vi "CRYFlatten Data Read.vi"(6 "error in":errorcluster, 9 "Path In":path) -> (0 "error out":errorcluster, 2 "Flatten Data Out":string, 3 "Path Out":path)   [LabVIEW 2013]
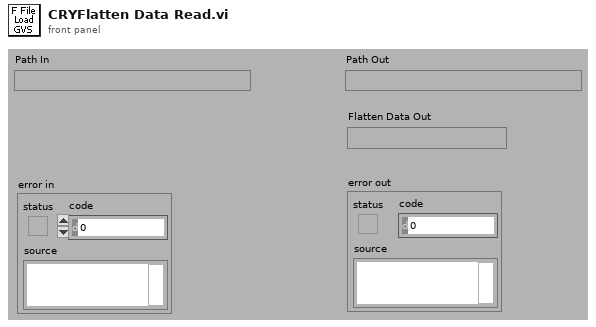
[diagram p1: front panel]
types:
  T1 = enum16{"open", "replace", "create", "open or create", "replace or create", "replace or create with confirmation"}
  T2 = enum16{"big-endian, network order", "native, host order", "little-endian"}
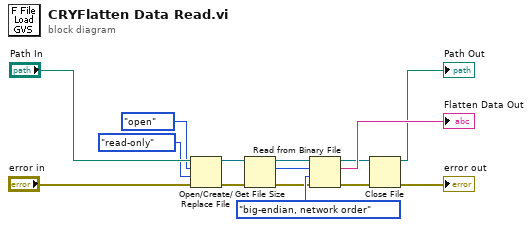
[diagram p0: block diagram]
diagram:
  n1 = Open/Create/Replace File(file path (use dialog)="Path In", error in="error in", operation (0:open)=T1."open", access (0:read/write)=enum16{"read/write", "read-only", "write-only"}."read-only") -> (refnum out=w6:refnum<file>, error out=w4:errorcluster)  [unwired: 3 out]
  n2 = Get File Size(file=w6, error in=w4) -> (refnum out=w5:refnum<file>, size (in bytes)=w2:i64, 0:w3:errorcluster)
  n3 = Read from Binary File(8:w3, 9:T2."big-endian, network order" ("Byte Order"), 10:w2, 11:w5) -> (0:w7:errorcluster, 2:→"Flatten Data Out":string, 3:w8:refnum<file>)  [unwired: 3 out]
  n4 = Close File(refnum=w8, error in=w7) -> (path=→"Path Out":path, error out=→"error out":errorcluster)
